vi "svc_Check dt for Equal Sample Rates.vi"(8 "error in (no error)":errorcluster, 10 "dt Y":dbl, 11 "dt X":dbl) -> (0 "error out":errorcluster, 3 "dt Y":dbl)   [LabVIEW 2017]
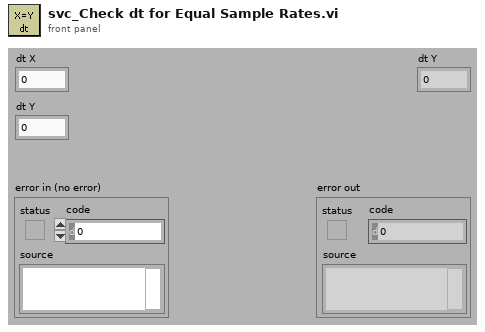
[diagram p1: front panel]
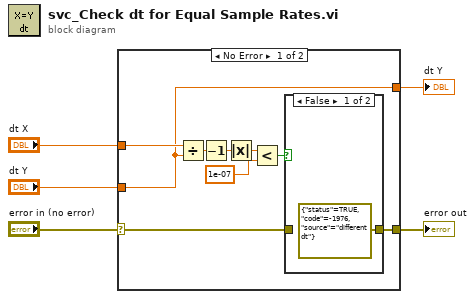
[diagram p0: block diagram]
diagram:
  n1 = case shown="No Error" "error in (no error)" {
    selector: "error in (no error)" -> [w9 w18]
    tunnel: "dt X" -> [w7 _]
    tunnel: "dt Y" -> [w6 w17]
    tunnel: [w8 w18] -> w2
    tunnel: [w6 w17] -> w1
    frame No Error {
      n2 = Divide(x=w7, y=w6) -> (x/y=w14:dbl)
      n3 = Decrement(x=w14) -> (x-1=w13:dbl)
      n4 = Absolute Value(x=w13) -> (abs(x)=w12:dbl)
      n5 = Less?(x=w12, y=1e-07) -> (x < y?=w11:bool)
      n6 = case shown="False" w11 {
        tunnel: w9 -> [_ w16]
        tunnel: [errorcluster {"status"=TRUE, "code"=-1976, "source"="different dt"} ("error IO") w16] -> w8
        frame False {
        }
        frame True {
        }
      }
    }
    frame Error {
    }
  }
  "error out" <- w2
  "dt Y" <- w1
